vi "controlOutput.vi"(7 "Set":bool, 8 "error in":errorcluster, 9 "enable output in":bool=TRUE, 10 "axis in":u8, 11 "connection ID":refnum<k5>) -> (0 "error out":errorcluster, 1 "enable output out":bool=TRUE, 2 "axis out":u8, 3 "connection ID":refnum<k5>)   [LabVIEW 2016]
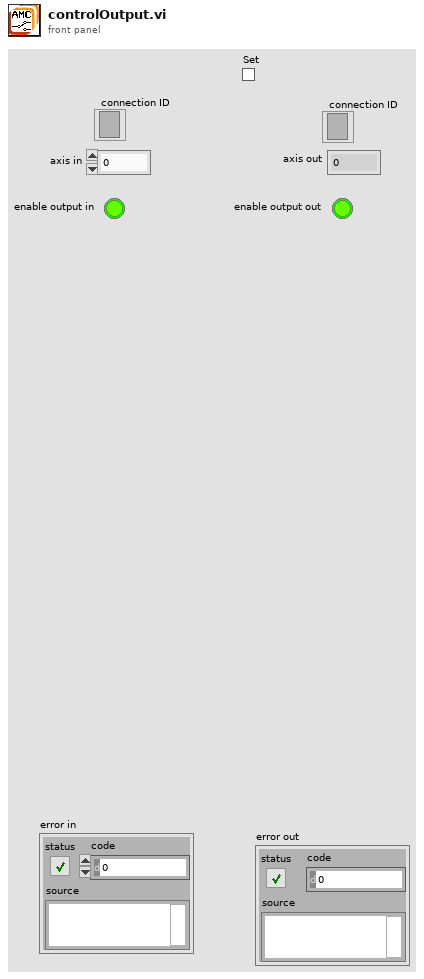
[diagram p1: front panel]
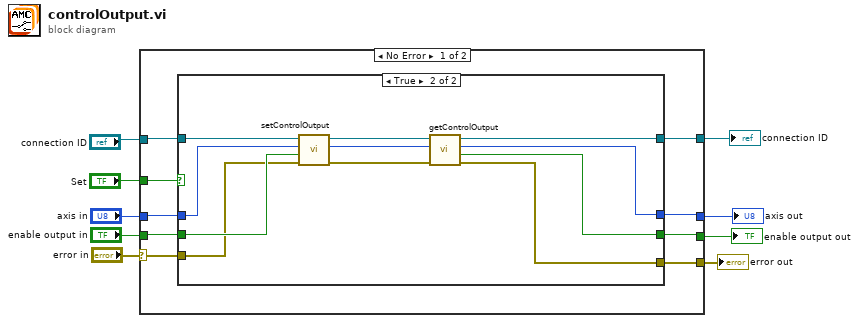
[diagram p0: block diagram]
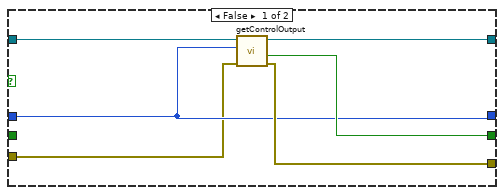
[diagram p2: hidden frame]
diagram:
  n1 = case shown="No Error" "error in" {
    selector: "error in" -> [w10 w39]
    tunnel: "axis in" -> [w16 w37]
    tunnel: [w11 w39] -> w1
    tunnel: [w15 w37] -> w8
    tunnel: "Set" -> [w12 _]
    tunnel: [w13 w38] -> w6
    tunnel: "enable output in" -> [w14 w38]
    tunnel: [w18 w36] -> w4
    tunnel: "connection ID" -> [w17 w36]
    frame No Error {
      n2 = case shown="True" w12 {
        tunnel: [w23 w31] -> w18
        tunnel: w17 -> [w24 w35]
        tunnel: w16 -> [w20 w28]
        tunnel: [w20 w26] -> w15
        tunnel: [w21 w25] -> w13
        tunnel: w14 -> [_ w34]
        tunnel: [w22 w27] -> w11
        tunnel: w10 -> [w19 w33]
        frame False {
          n3 = call "getControlOutput.vi"("error in"=w19, "axis"=w20, "connection ID"=w24) -> ("error out"=w22:errorcluster, "boolean"=w21:bool, "connection ID"=w23:refnum<k5>)  [unwired: 5 in, 1 out]
        }
        frame True {
          n4 = call "setControlOutput.vi"("error in"=w33, "enable"=w34, "axis"=w28, "connection ID"=w35) -> ("error out"=w30:errorcluster, "axis_out"=w29:i32, "connection ID"=w32:refnum<k5>)  [unwired: 5 in]
          n5 = call "getControlOutput.vi"("error in"=w30, "axis"=w29, "connection ID"=w32) -> ("error out"=w27:errorcluster, "boolean"=w25:bool, "axis_out"=w26:i32, "connection ID"=w31:refnum<k5>)  [unwired: 5 in]
        }
      }
    }
    frame Error {
    }
  }
  "error out" <- w1
  "axis out" <- w8
  "enable output out" <- w6
  "connection ID" <- w4
